vi "Command Wait.vi"(7 "Startup":bool, 11 "Time to Wait (ms)":dbl) -> (1 "Right Wheel":dbl, 2 "Left Wheel":dbl, 4 "Reint":bool, 6 "Completed":bool)   [LabVIEW 2017]
uses:
  Command Execution State.ctl
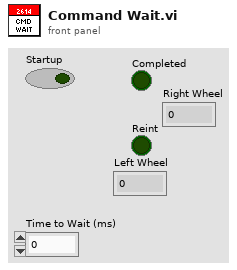
[diagram p1: front panel]
types:
  T1 = typedef "Command Execution State.ctl" = enum16{"Initialize", "Execute", "Finish"}
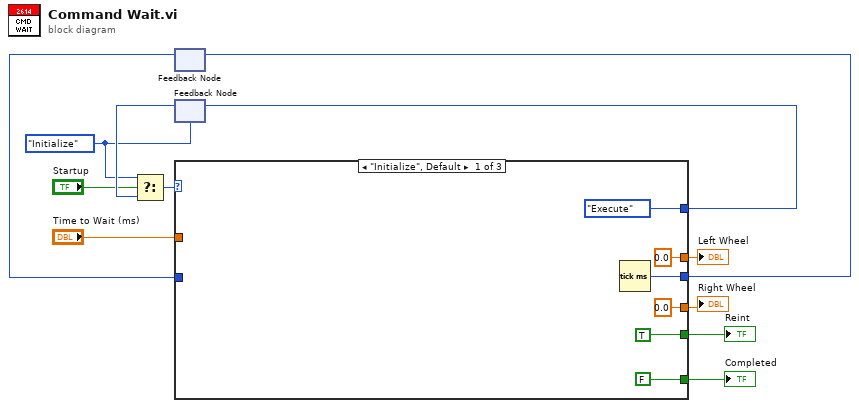
[diagram p0: block diagram]
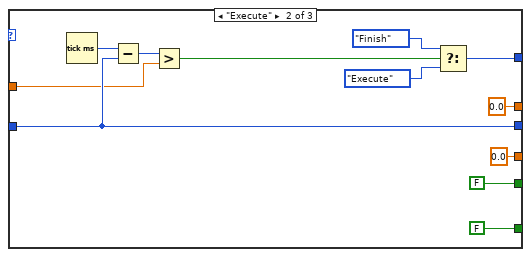
[diagram p2: hidden frame]
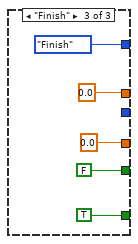
[diagram p3: hidden frame]
diagram:
  w9 = Command_Execution_State."Initialize" ("Play State")
  n1 = feedback #1() -> (w4:u32)  [unwired: 1 in]
  n2 = feedback #2(w9) -> (w10:T1)
  n3 = Select(t=w9, s="Startup", f=w10) -> (s? t:f=w12:T1)
  n4 = case shown="\"Initialize\", Default" w12 {
    tunnel: [Command_Execution_State."Execute" ("Play State") w21 Command_Execution_State."Finish" ("Play State")] -> w11
    tunnel: [FALSE FALSE TRUE] -> w6
    tunnel: [TRUE FALSE FALSE] -> w7
    tunnel: [w15 w26 _] -> w5
    tunnel: w4 -> [_ w26 _]
    tunnel: "Time to Wait (ms)" -> [_ w25 _]
    tunnel: [0.0 0.0 0.0] -> w1
    tunnel: [0.0 0.0 0.0] -> w2
    frame "Initialize", Default {
      n5 = Tick Count (ms)() -> (millisecond timer value=w15:u32)
    }
    frame "Execute" {
      n6 = Tick Count (ms)() -> (millisecond timer value=w28:u32)
      n7 = Subtract(x=w28, y=w26) -> (x-y=w27:u32)
      n8 = Greater?(x=w27, y=w25) -> (0:w22:bool)
      n9 = Select(t=Command_Execution_State."Finish" ("Play State"), s=w22, f=Command_Execution_State."Execute" ("Play State")) -> (s? t:f=w21:T1)
    }
    frame "Finish" {
    }
  }
  "Reint" <- w7
  "Completed" <- w6
  "Right Wheel" <- w2
  "Left Wheel" <- w1
  n10 = feedback-in #1(w5) -> ()
  n11 = feedback-in #2(w11) -> ()
